vi "Ctor.vi"(8 "error in (no error)":errorcluster, 11 "ColumnPanel in":refnum<class "ColumnPanel.lvclass">) -> (0 "error out":errorcluster, 3 "ColumnPanel out":refnum<class "ColumnPanel.lvclass">)   [LabVIEW 2020, in "Conditum-Tools.lvlib" / "ColumnPanel.lvclass"]
uses:
  ColumnPanel.lvclass
  Conditum-Clone/Columns/Type/Type.lvclass
  ColumnPanel.lvclass/ColumnPanel.ctl
  <vilib>/IlluminatedG/IG OOPanel/OOPanel/ArrayPanel/ArrayPanel.lvclass
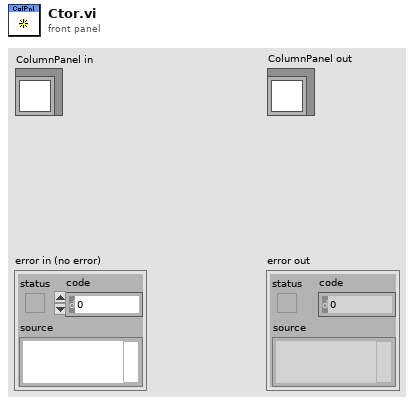
[diagram p1: front panel]
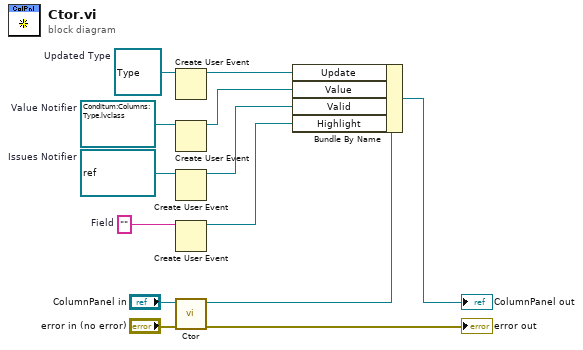
[diagram p0: block diagram]
diagram:
  w2 = ""  # Field
  w4 = refnum<notifier> refnum  # Issues Notifier
  w6 = refnum<notifier> refnum  # Value Notifier
  w8 = refnum<class "Type.lvclass"> refnum  # Updated Type
  n1 = Create User Event(user event datatype=w8) -> (user event=w7:refnum<user-event>)  [unwired: 1 in, 1 out]
  n2 = Create User Event(user event datatype=w6) -> (user event=w5:refnum<user-event>)  [unwired: 1 in, 1 out]
  n3 = Create User Event(user event datatype=w4) -> (user event=w3:refnum<user-event>)  [unwired: 1 in, 1 out]
  n4 = Create User Event(user event datatype=w2) -> (user event=w1:refnum<user-event>)  [unwired: 1 in, 1 out]
  n5 = call-parent "Ctor.vi"("error in (no error)"="error in (no error)", "ArrayPanel in"="ColumnPanel in") -> ("error out"=→"error out":errorcluster, "ArrayPanel out"=w11:refnum<class "ColumnPanel.lvclass">)  [unwired: 8 in]
  n6 = Bundle By Name(cluster=w11, "Update"=w7, "Value"=w5, "Valid"=w3, "Highlight"=w1) -> (→"ColumnPanel out":refnum<class "ColumnPanel.lvclass">)
